vi "Identify.vi"(8 "error in (no error)":errorcluster, 11 "IIP3 Calculation in":refnum<class "IIP3Calculation.lvclass">) -> (0 "error out":errorcluster, 2 "Plugin is Valid":bool, 3 "IIP3 Calculation out":refnum<class "IIP3Calculation.lvclass">)   [LabVIEW 2018, in "IIP3Calculation.lvlib" / "IIP3Calculation.lvclass"]
uses:
  IIP3Calculation.lvclass
  C:/Sequence Automation/Plugins/Measurement Interface.lvlibp/Measurement Interface.lvclass
  Plugins/Measurement Interface.lvlibp/Private Methods/Measurement Definition Entry/Read Measurement Definition Entry.vi
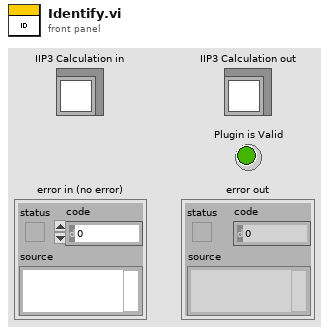
[diagram p1: front panel]
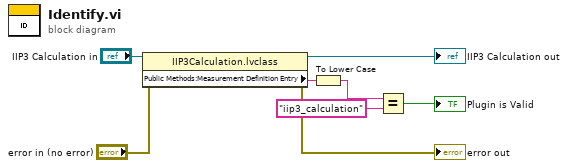
[diagram p0: block diagram]
diagram:
  n1 = property class="IIP3Calculation.lvclass"(reference="IIP3 Calculation in", error in="error in (no error)") -> (reference out=→"IIP3 Calculation out":refnum<class "IIP3Calculation.lvclass">, error out=→"error out":errorcluster, "Public Methods:Measurement Definition Entry"=w4:string)
  n2 = To Lower Case(string=w4) -> (all lower case string=w3:string)
  n3 = Equal?(x=w3, y="iip3_calculation") -> (x = y?=→"Plugin is Valid":bool)
